vi "Get configuration chain.vi"(8 "error in (no error)":errorcluster, 11 "BMCBase in":refnum<class "BMC.lvclass">) -> (0 "error out":errorcluster, 1 "class name":string[](array[string]), 2 "configuration chain":variant[](array[variant]), 3 "BMCBase out":refnum<class "BMC.lvclass">)   [LabVIEW 2012, in "BMC.lvclass"]
doc: "Returns an array of variants containing the configuration clusters of each class in the inheritance chain (lowest child class first), together with an array of all class names in the inheritance chain.\n\nFor classes without configuration cluster, the configuration chain contains empty variants."
uses:
  BMC.lvclass
  Murmex/LabVIEW/Murmex/Murmex/Murmex.lvclass
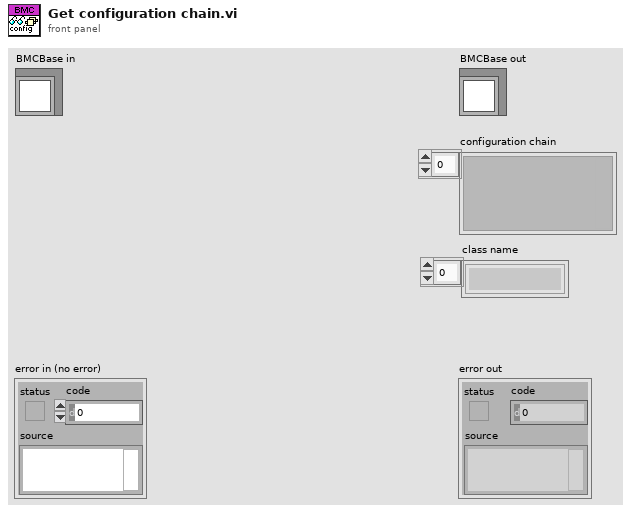
[diagram p1: front panel]
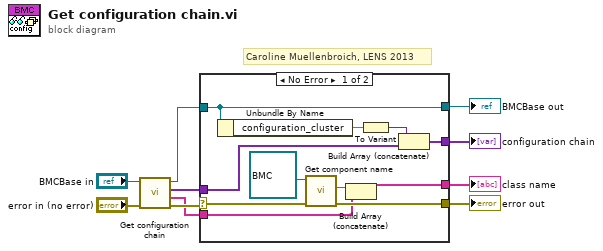
[diagram p0: block diagram]
diagram:
  # "Caroline Muellenbroich, LENS 2013"
  n1 = call-parent "Get configuration chain.vi"("error in (no error)"="error in (no error)", "MurmexBase in"="BMCBase in") -> ("error out"=w9:errorcluster, "class name"=w5:string[], "configuration chain"=w2:variant[], "MurmexBase out"=w3:refnum<class "BMC.lvclass">)  [unwired: 6 in]
  n2 = case shown="No Error" w9 {
    selector: w9 -> [w18 w25]
    tunnel: [w17 w25] -> w8
    tunnel: w3 -> [w13 w24]
    tunnel: [w13 w24] -> w6
    tunnel: w5 -> [w15 w22]
    tunnel: [w14 w22] -> w4
    tunnel: w2 -> [w12 w23]
    tunnel: [w11 w23] -> w1
    frame No Error {
      n3 = Unbundle By Name(w13) -> ("configuration_cluster"=w21)
      n4 = call "Get component name.vi"("error in (no error)"=w18, "Murmex in"=refnum<class "BMC.lvclass"> refnum ("BMC")) -> ("error out"=w17:errorcluster, "component name"=w16:string)  [unwired: 7 in, 1 out]
      n5 = Build Array (concatenate)(w16, w15) -> (w14:string[])
      n6 = To Variant(anything=w21) -> (Variant=w20:variant)
      n7 = Build Array (concatenate)(w20, w12) -> (w11:variant[])
    }
    frame Error {
    }
  }
  "error out" <- w8
  "BMCBase out" <- w6
  "configuration chain" <- w1
  "class name" <- w4
